vi "FTW-Request-Construct.vi"(5 "Verbatim Request":string, 7 "Response Broker":refnum<queue>, 11 "error in":errorcluster) -> (4 "FTW Request out":refnum<class "FTW-Request.lvclass">, 15 "error out":errorcluster)   [LabVIEW 2012, in "FTW-Actor.lvlib" / "FTW-Request.lvclass"]
uses:
  FTW-Request.lvclass
  FTW-Request.lvclass/FTW-Request.ctl
panel:
  # "Inputs"
  # "Outputs"
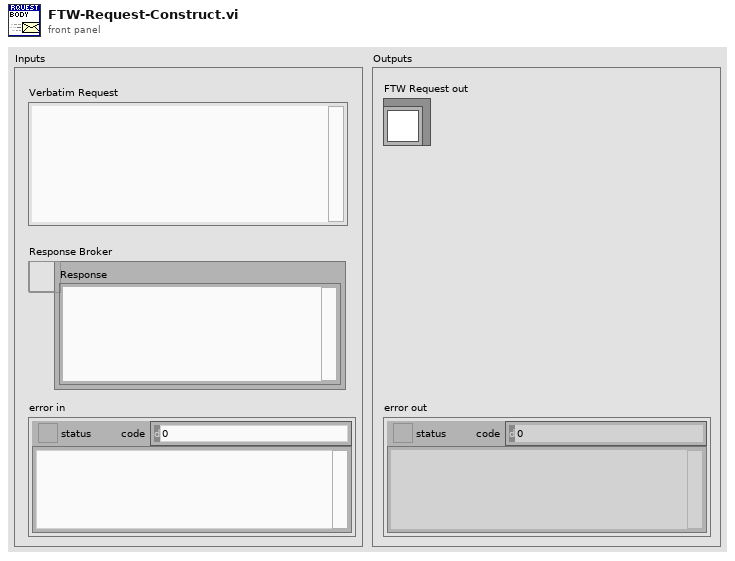
[diagram p1: front panel]
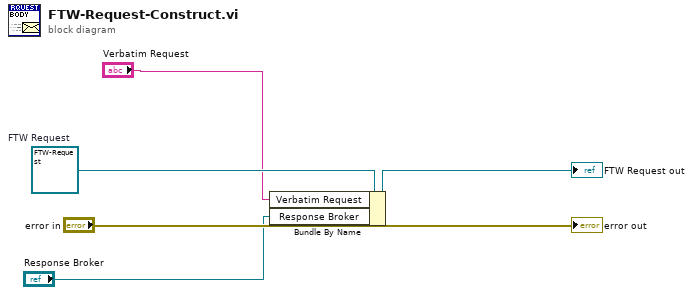
[diagram p0: block diagram]
diagram:
  w5 = refnum<class "FTW-Request.lvclass"> refnum  # FTW Request
  n1 = Bundle By Name(cluster=w5, "Verbatim Request"="Verbatim Request", "Response Broker"="Response Broker") -> (→"FTW Request out":refnum<class "FTW-Request.lvclass">)
  "error out" <- "error in"
